vi "Igor_LoadLargeWaveUsingFile.vi"(7 "Path":path, 8 "error in":errorcluster, 9 "Wave":dbl[](array[numeric]), 10 "Wavename":string, 11 "Application":refnum<k7>) -> (0 "error out":errorcluster, 3 "Application":refnum<k7>)   [LabVIEW 2019]
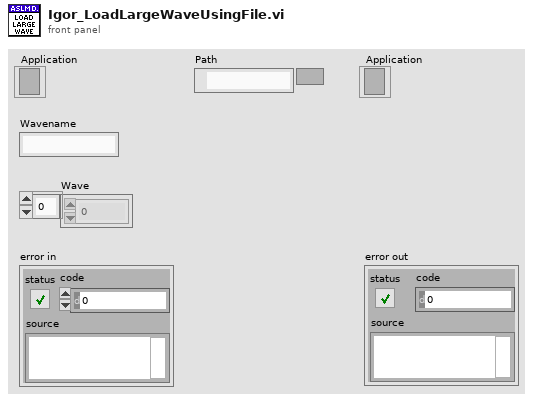
[diagram p1: front panel]
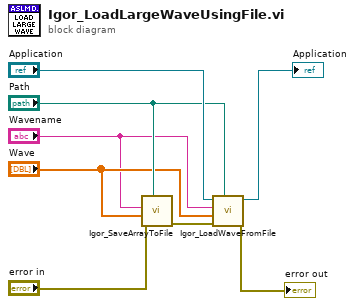
[diagram p0: block diagram]
diagram:
  n1 = call "Igor_SaveArrayToFile.vi"("Path"="Path", "error in (no error)"="error in", "Wave"="Wave", "Wavename"="Wavename") -> ("error out"=w6:errorcluster)  [unwired: 6 in, 1 out]
  n2 = call "Igor_LoadWaveFromFile.vi"("Path"="Path", "error in (no error)"=w6, "Wave"="Wave", "Wavename"="Wavename", "Application"="Application") -> ("error out"=→"error out":errorcluster, "Application"=→"Application":refnum<k7>)  [unwired: 5 in]
